vi "_parse Log Line.vi"(11 "String":string) -> (0 "LogType":string, 2 "State":string, 3 "CSM":string)   [LabVIEW 2017, in "csm-tool-support.lvlib"]
uses:
  csm-tool-support.lvlib
  _Shared/CSM Shared.lvlib
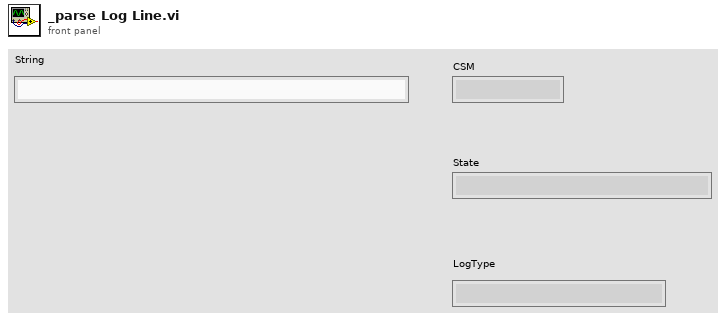
[diagram p1: front panel]
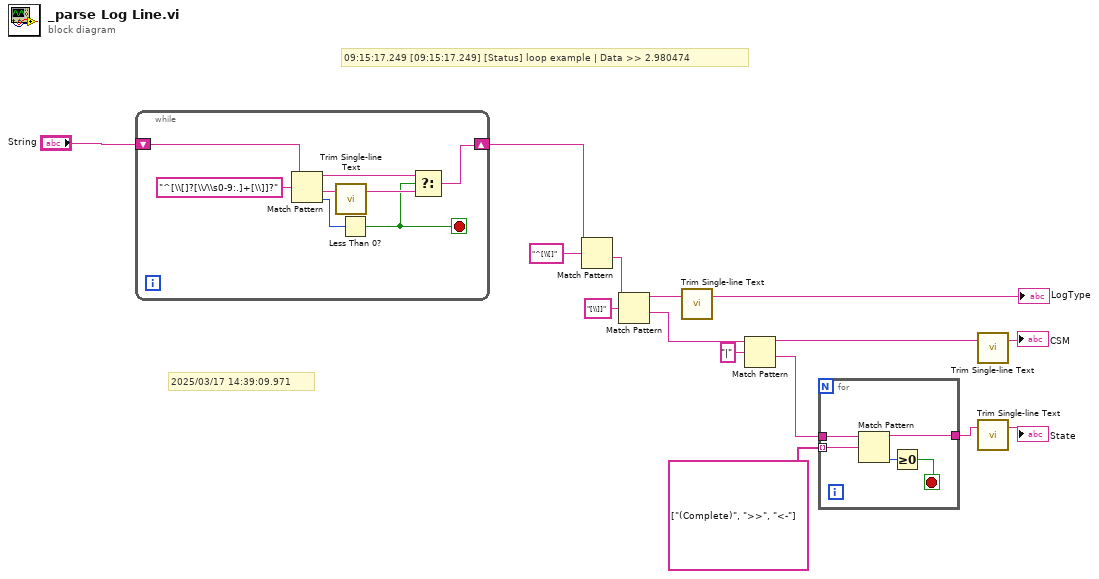
[diagram p0: block diagram]
diagram:
  # "09:15:17.249 [09:15:17.249] [Status] loop example | Data >> 2.980474"
  # "2025/03/17 14:39:09.971"
  n1 = while {
    shift-right: [w16] -> w14
    shift-left: "String" -> [w21]
    stop <- w17 stop-if-true
    n2 = Match Pattern(string=w21, regular expression="^[\\[]?[\\/\\s0-9:.]+[\\]]?") -> (before substring=w19:string, after substring=w22:string, offset past match=w20:i32)  [unwired: 1 in, 1 out]
    n3 = call "Trim Single-line Text.vi"("single-line text"=w22) -> ("trimed text"=w18:string)  [unwired: 2 in]
    n4 = Less Than 0?(x=w20) -> (x < 0?=w17:bool)
    n5 = Select(t=w19, s=w17, f=w18) -> (s? t:f=w16:string)
  }
  n6 = Match Pattern(string=w14, regular expression="^[\\[]") -> (after substring=w12:string)  [unwired: 1 in, 3 out]
  n7 = Match Pattern(string=w12, regular expression="[\\]]") -> (before substring=w11:string, after substring=w8:string)  [unwired: 1 in, 2 out]
  n8 = call "Trim Single-line Text.vi"("single-line text"=w11) -> ("trimed text"=→"LogType":string)  [unwired: 2 in]
  n9 = Match Pattern(string=w8, regular expression="|") -> (before substring=w4:string, after substring=w6:string)  [unwired: 1 in, 2 out]
  n10 = for {
    tunnel: w6 -> [w28]
    tunnel: string[] ["(Complete)", ">>", "<-"] ("regular expression") -> [w27] mode=indexing
    tunnel: [w26] -> w2
    stop <- w24 stop-if-true
    n11 = Match Pattern(string=w28, regular expression=w27) -> (before substring=w26:string, offset past match=w25:i32)  [unwired: 1 in, 2 out]
    n12 = Greater Or Equal To 0?(x=w25) -> (x >= 0?=w24:bool)
  }
  n13 = call "Trim Single-line Text.vi"("single-line text"=w4) -> ("trimed text"=→"CSM":string)  [unwired: 2 in]
  n14 = call "Trim Single-line Text.vi"("single-line text"=w2) -> ("trimed text"=→"State":string)  [unwired: 2 in]
